vi "Auto_Conf.vi"() -> ()   [LabVIEW 2012]
panel:
  in  "Has Turned":bool
  in  "AutoToRun":u8
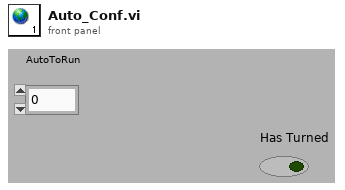
[diagram p1: front panel]
diagram:
